vi "CoboltLaser_ResponseCheck.vi"(0 "Response":string, 1 "ExpectedResponseType":T1, 2 "ExpectedResponseMinimumLength":i32 min=0 step=1, 3 "ErrorMessage":string, 4 "GenerateErrorIfFail":bool, 5 "ErrorIn":errorcluster, 6 "Display Error message":bool, 7 "i":i32) -> (15 "ResponseOK":bool, 16 "Retry":bool, 19 "ErrorOut":errorcluster)   [LabVIEW 2019]
doc: "Use this template to build a VI to use as a subVI."
uses:
  <userlib>/CoboltLaser/CoboltLaser_Controls/ExpectedResponseType.ctl
  Instance           1 26Saved   PR59_ResponseCheck .vi
  <vilib>/regexp/Match Regular Expression.xnode
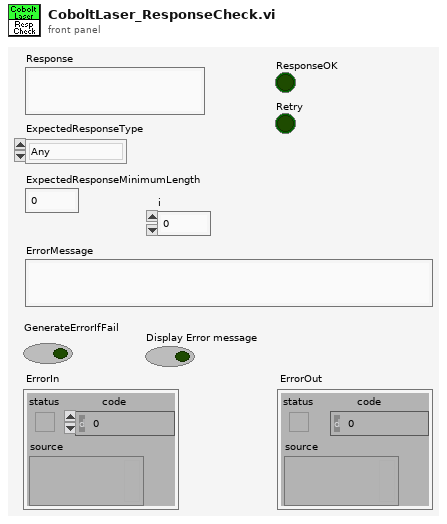
[diagram p1: front panel]
types:
  T1 = typedef "ExpectedResponseType.ctl" = enum16{"Any", "Digits Only", "Non-Digits Only"}
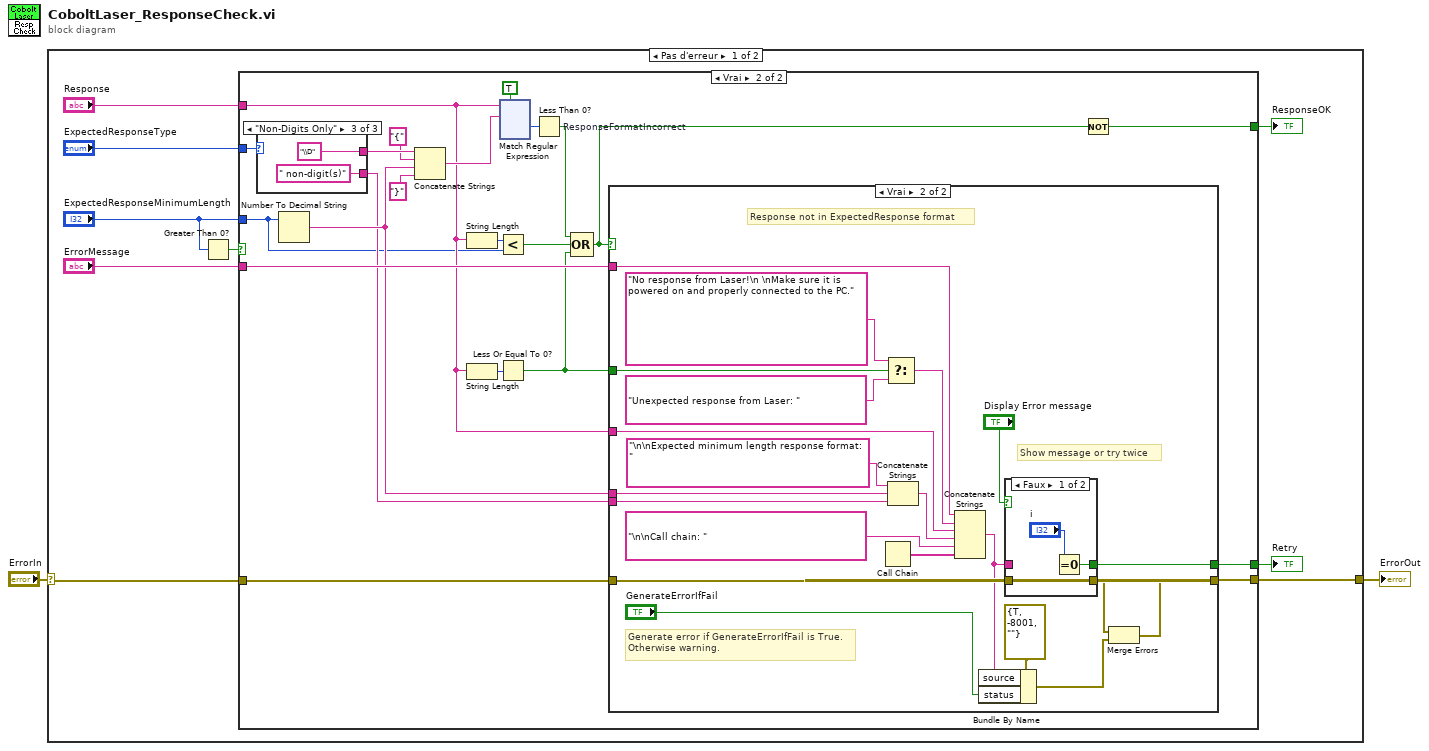
[diagram p0: block diagram]
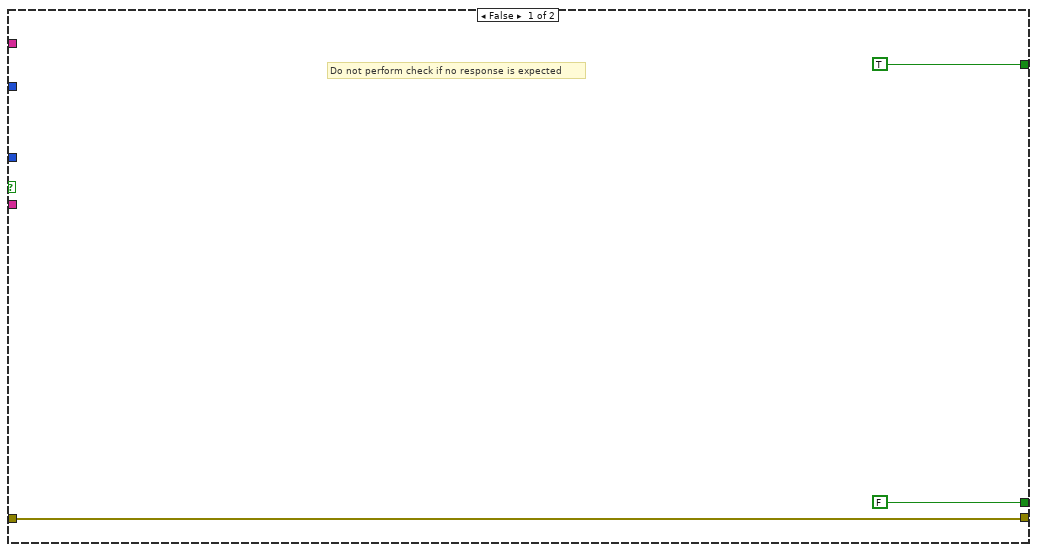
[diagram p2: hidden frame]
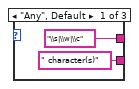
[diagram p3: hidden frame]
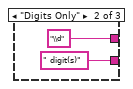
[diagram p4: hidden frame]
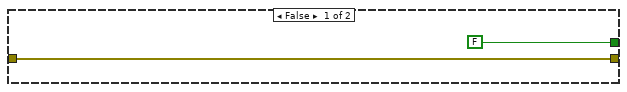
[diagram p5: hidden frame]
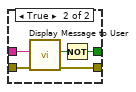
[diagram p6: hidden frame]
diagram:
  n1 = case shown="Pas d'erreur" "ErrorIn" {
    selector: "ErrorIn" -> [w9 w185]
    tunnel: [w11 w185] -> w1
    frame No Error {
      n2 = Greater Than 0?(x="ExpectedResponseMinimumLength") -> (x > 0?=w3:bool)
      n3 = case shown="Vrai" w3 {
        tunnel: [w12 w15] -> w11
        tunnel: "ErrorMessage" -> [_ w36]
        tunnel: w9 -> [w12 w35]
        tunnel: [FALSE w34] -> w8
        tunnel: "Response" -> [_ w20]
        tunnel: "ExpectedResponseType" -> [_ w30]
        tunnel: "ExpectedResponseMinimumLength" -> [_ w18]
        tunnel: [TRUE w24] -> w4
        frame False {
          # "Do not perform check if no response is expected"
        }
        frame True {
          n4 = case shown="\"Non-Digits Only\"" w30 {
            tunnel: ["\\s|\\w|\\c" "\\d" "\\D"] -> w29
            tunnel: [" character(s)" " digit(s)" " non-digit(s)"] -> w22
            frame "Any", Default {
            }
            frame "Digits Only" {
            }
            frame "Non-Digits Only" {
            }
          }
          n5 = Number To Decimal String(number=w18) -> (decimal integer string=w23:string)  [unwired: 1 in]
          n6 = Concatenate Strings(w29, "{", w23, "}") -> (w26:string)
          n7 = String Length(string=w20) -> (length=w19:i32)
          n8 = String Length(string=w20) -> (length=w33:i32)
          n9 = Less?(x=w19, y=w18) -> (x < y?=w16:bool)
          n10 = Less Or Equal To 0?(x=w33) -> (x <= 0?=w17:bool)
          n11 = xnode "Match Regular Expression"("input string"=w20, "regular expression"=w26, "ignore case? (F)"=TRUE) -> ("offset past match"=w32:i32)  [unwired: 3 in, 4 out]
          n12 = Less Than 0? "ResponseFormatIncorrect"(x=w32) -> (x < 0?=w31:bool)
          n13 = Compound Arithmetic op=OR(w31, w16, w17) -> (w25:bool)
          n14 = case shown="Vrai" w25 {
            tunnel: [w155 w159] -> w15
            tunnel: w35 -> [w155 w175]
            tunnel: w20 -> [_ w172]
            tunnel: w36 -> [_ w173]
            tunnel: [FALSE w156] -> w34
            tunnel: w17 -> [_ w171]
            tunnel: w23 -> [_ w164]
            tunnel: w22 -> [_ w162]
            frame False {
            }
            frame True {
              # "Show message or try twice"
              # "Response not in ExpectedResponse format"
              # "Generate error if GenerateErrorIfFail is True.\nOtherwise warning."
              n15 = Call Chain() -> (call chain=w168:string[])
              n16 = Select(t="No response from Laser!\n \nMake sure it is powered on and properly connected to the PC." ("Message"), s=w171, f="Unexpected response from Laser: " ("Message")) -> (s? t:f=w167:string)
              n17 = Concatenate Strings("\n\nExpected minimum length response format: " ("Message"), w164, w162) -> (w163:string)
              n18 = Concatenate Strings(w173, w167, w172, w163, "\n\nCall chain: " ("Message"), w168) -> (w174:string)
              n19 = Bundle By Name(cluster=errorcluster {"status"=TRUE, "code"=-8001, "source"=""} ("error out"), "source"=w174, "status"="GenerateErrorIfFail") -> (w160:errorcluster)
              n20 = case shown="Faux" "Display Error message" {
                tunnel: w175 -> [w179 w184]
                tunnel: w174 -> [_ w183]
                tunnel: [w178 w180] -> w156
                tunnel: [w179 w182] -> w161
                frame False {
                  n21 = Equal To 0?(x="i") -> (x = 0?=w178:bool)
                }
                frame True {
                  n22 = call "Display Message to User"("error in (no error)"=w184, "Message"=w183) -> ("error out"=w182:errorcluster, "Continue"=w181:bool)  [unwired: 1 in, 7 out]
                  n23 = Not(x=w181) -> (.not. x?=w180:bool)
                }
              }
              n24 = Merge Errors(w161, w160) -> (w159:errorcluster)
            }
          }
          n25 = Not(x=w25) -> (.not. x?=w24:bool)
        }
      }
      "ResponseOK" <- w4
      "Retry" <- w8
    }
    frame Error {
    }
  }
  "ErrorOut" <- w1
